vi "Main.vi"(8 "error in":errorcluster, 9 "Error Queue":refnum<queue>, 11 "Application Events":refnum<user-event>) -> (0 "error out":errorcluster)   [LabVIEW 2020, in "Sensor Interface.lvlib"]
doc: "VI Template with default error structure"
uses:
  Sensor Interface.lvlib
  Error/Controls/Error Message Object.ctl
  Controller/Controls/Application Modules.ctl
  Error/Controls/Error Commands.ctl
  Controller/Controls/Application Event Object.ctl
  Controller/Controls/Application Events.ctl
  Controls/Event Loop Data.ctl
  Controls/Operational Loop Data.ctl
  Controls/Operational Loop Commands.ctl
  Controller/Controller.lvlib
  Error/Error Handler.lvlib
panel:
  in  "Funds Dispensed":bool
  in  "Deposit Received":bool
  # "[Covers: UI4] \n[Covers: UI4A] \n[Covers: UI4B]"
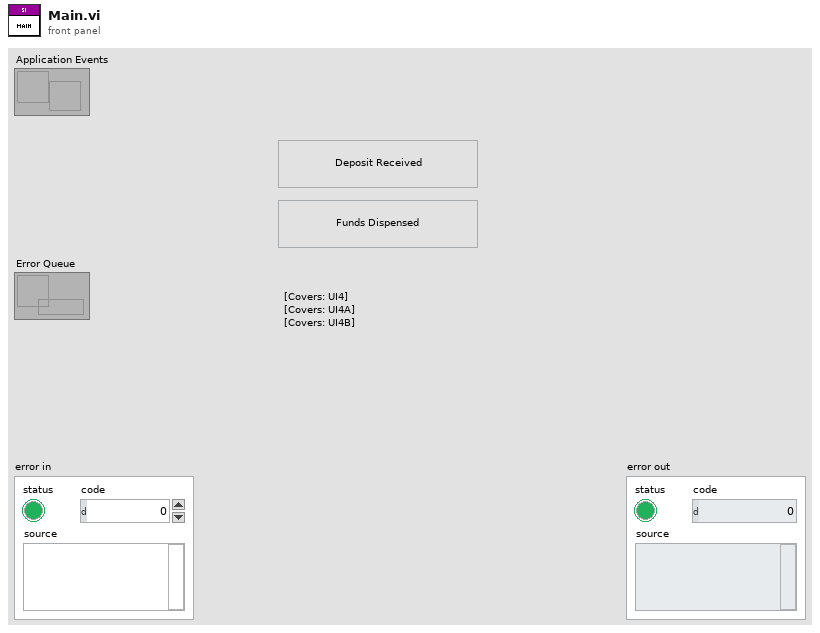
[diagram p1: front panel]
types:
  T1 = typedef "Sensor Interface.lvlib/Operational Loop Data.ctl" = cluster{"Current Module":T2}
  T2 = typedef "Controller.lvlib/Application Modules.ctl" = enum16{"Controller", "Error Module", "User Console", "Display Console", "Sensor Interface"}
  T3 = typedef "Sensor Interface.lvlib/Event Loop Data.ctl" = cluster{"Current Module":T2}
  T4 = typedef "Controller.lvlib/Application Events.ctl" = enum16{"Shutdown", "Initialize", "New Transaction", "Balance Inquiry", "Deposit", "Withdrawal", "Fast Cash 50$", "Terminate Session", "Login", "Verify Account"}
  T5 = typedef "Sensor Interface.lvlib/Operational Loop Commands.ctl" = enum16{"Shutdown"}
  T6 = enum16{"Load References", "Release References", "Get References"}
  T7 = typedef "Controller.lvlib/Controller Message Object.ctl" = cluster{"Commands":T8, "Source Module":T2, "Event Data":variant}
  T8 = typedef "Controller Commands.ctl" = enum16{"Shutdown"}
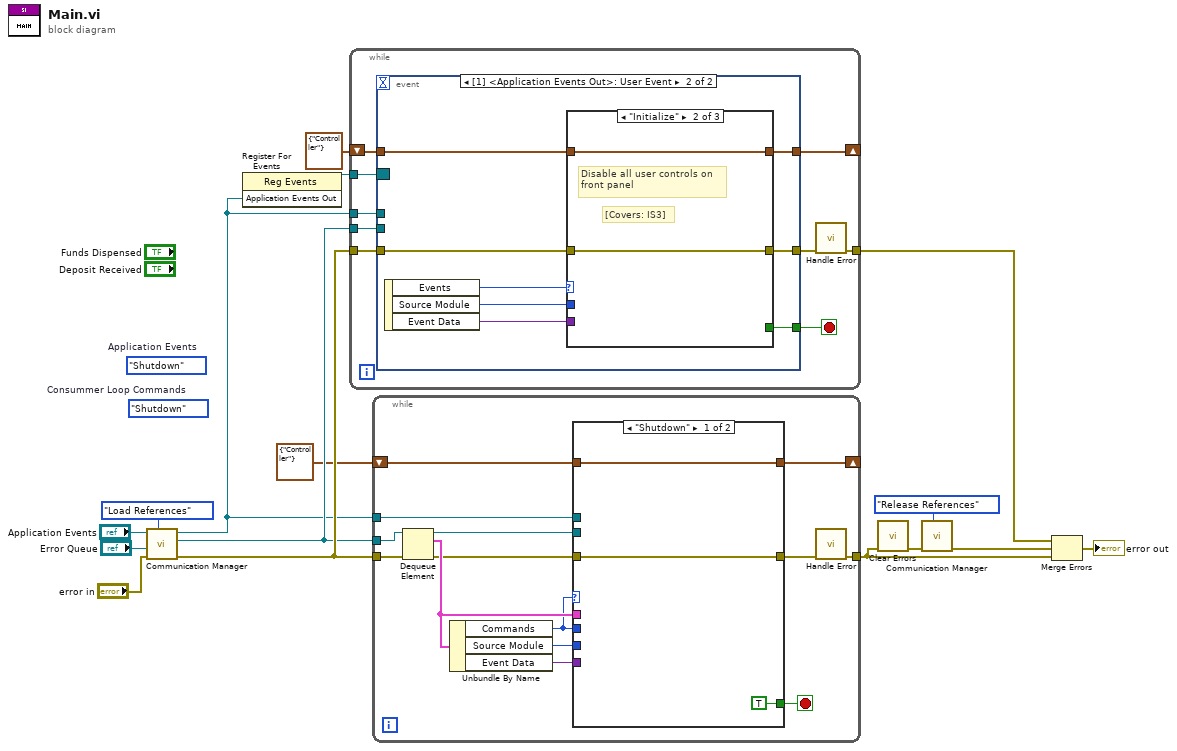
[diagram p0: block diagram]
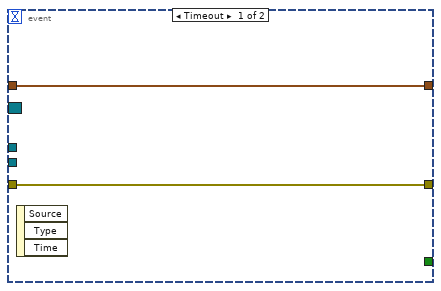
[diagram p3: hidden frame]
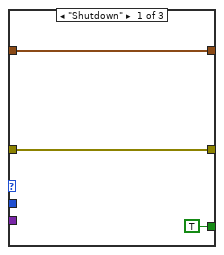
[diagram p4: hidden frame]
diagram:
  (unwired) Application_Events."Shutdown"  # Application Events
  (unwired) Operational_Loop_Commands."Shutdown"  # Consummer Loop Commands
  n1 = call "Communication Manager.vi"("Mode"=T6."Load References", "error in"="error in", "Error Queue"="Error Queue", "Application Events"="Application Events") -> ("error out"=w13:errorcluster, "Module Queue Out"=w5:refnum<queue>, "Application Events Out"=w4:refnum<user-event>)  [unwired: 4 in, 1 out]
  n2 = register-events(w4) -> (reference out=w3:refnum<event-registration>)  [unwired: 2 in, 1 out]
  n3 = while {
    tunnel: w13 -> [w24]
    tunnel: w4 -> [w23]
    tunnel: [w25] -> w11
    tunnel: w5 -> [w22]
    tunnel: w3 -> [w21]
    shift-right: [w18] -> _
    shift-left: T3 {"Current Module"=enum."Controller"} ("Event Loop Data") -> [w17]
    stop <- w19 stop-if-true
    n4 = event shown="[1] <Application Events Out>: User Event" {
      selector: w21 -> [_ _]
      dyn-events: _ -> [_ _]
      timeout: _ -> [_ _]
      tunnel: w24 -> [w27 w34]
      tunnel: w23 -> [_ _]
      tunnel: w22 -> [_ _]
      tunnel: [w27 w35] -> w20
      tunnel: [_ w30] -> w19
      tunnel: [w26 w29] -> w18
      tunnel: w17 -> [w26 w28]
      event Timeout {
        n5 = event-data() -> ()  [unwired: 1 in, 3 out]
      }
      event User Event {
        n6 = event-data() -> ("Events"=w33:T4, "Source Module"=w32:T2, "Event Data"=w31:variant)  [unwired: 1 in]
        n7 = case shown="\"Initialize\"" w33 {
          tunnel: [w38 w40 w42] -> w35
          tunnel: w34 -> [w38 w40 w42]
          tunnel: w32 -> [_ _ _]
          tunnel: w31 -> [_ _ _]
          tunnel: [TRUE _ _] -> w30
          tunnel: [w36 w39 w41] -> w29
          tunnel: w28 -> [w36 w39 w41]
          frame "Shutdown" {
          }
          frame "Initialize" {
            # "[Covers: IS3]"
            # "Disable all user controls on \nfront panel"
          }
          frame Default {
          }
        }
      }
    }
    n8 = call "Handle Error.vi"("error in"=w20) -> ("error out"=w25:errorcluster)  [unwired: 10 in]
  }
  n9 = while {
    tunnel: w13 -> [w55]
    tunnel: w5 -> [w54]
    tunnel: [w56] -> w7
    tunnel: w4 -> [w47]
    shift-right: [w44] -> _
    shift-left: T1 {"Current Module"=enum."Controller"} ("Operational Loop Data") -> [w45]
    stop <- w48 stop-if-true
    n10 = Dequeue Element(queue=w54, error in (no error)=w55) -> (queue out=w46:refnum<queue>, element=w52:T7, error out=w43:errorcluster)  [unwired: 1 in, 1 out]
    n11 = Unbundle By Name(w52) -> ("Commands"=w49:T8, "Source Module"=w51:T2, "Event Data"=w50:variant)
    n12 = case shown="\"Shutdown\"" w49 {
      tunnel: w43 -> [w59 w61]
      tunnel: [w59 w61] -> w53
      tunnel: w52 -> [_ _]
      tunnel: w49 -> [_ _]
      tunnel: w51 -> [_ _]
      tunnel: w50 -> [_ _]
      tunnel: [TRUE _] -> w48
      tunnel: w47 -> [_ _]
      tunnel: w46 -> [_ _]
      tunnel: w45 -> [w57 w60]
      tunnel: [w57 w60] -> w44
      frame "Shutdown" {
      }
      frame Default {
      }
    }
    n13 = call "Handle Error.vi"("error in"=w53) -> ("error out"=w56:errorcluster)  [unwired: 10 in]
  }
  n14 = call <vilib>:"Clear Errors.vi"("error in (no error)"=w7) -> ("error out"=w10:errorcluster)  [unwired: 5 in, 1 out]
  n15 = call "Communication Manager.vi"("Mode"=T6."Release References", "error in"=w10) -> ("error out"=w6:errorcluster)  [unwired: 6 in, 3 out]
  n16 = Merge Errors(w11, w6, w7) -> (→"error out":errorcluster)
